vi "All Windows Out.vi"(8 "error in (no error)":errorcluster, 11 "[MDI] Parent in":refnum<class "[MDI] Parent.lvclass">) -> (0 "error out":errorcluster, 3 "[MDI] Parent out":refnum<class "[MDI] Parent.lvclass">)   [LabVIEW 2020, in "[MDI] Parent.lvlib" / "[MDI] Parent.lvclass"]
uses:
  [MDI] Parent.lvclass
  [MDI] Parent.lvclass/[MDI] Parent.ctl
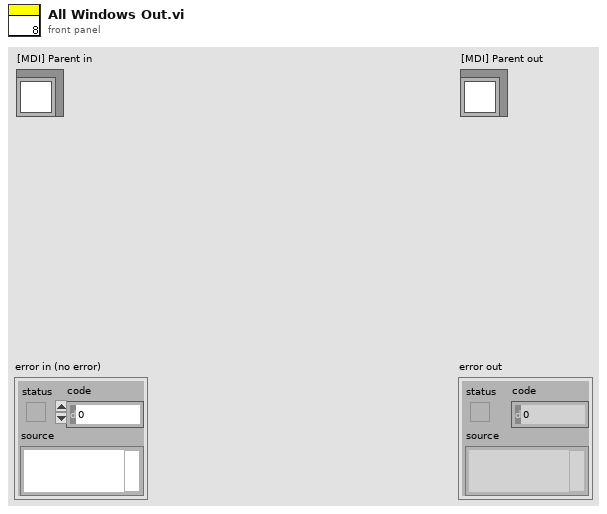
[diagram p1: front panel]
types:
  T1 = enum32{"Invalid", "Standard", "Closed", "Hidden", "Minimized", "Maximized"}
  T2 = typedef "LVRectTypeDef.ctl" = cluster{"Left":i16, "Top":i16, "Right":i16, "Bottom":i16}
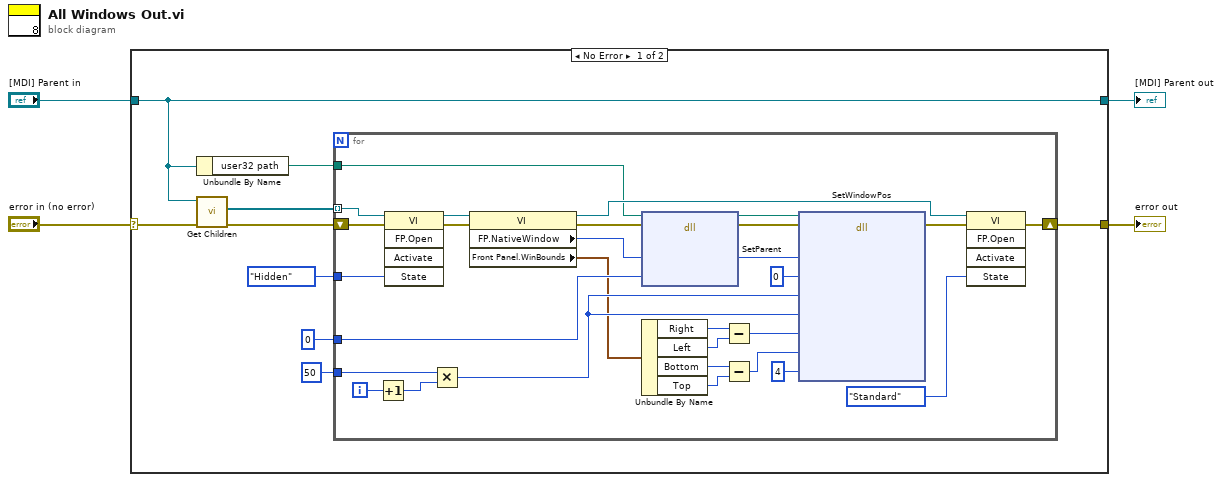
[diagram p0: block diagram]
diagram:
  n1 = case shown="No Error" "error in (no error)" {
    selector: "error in (no error)" -> [w13 w44]
    tunnel: [w7 w44] -> w3
    tunnel: [w6 w43] -> w1
    tunnel: "[MDI] Parent in" -> [w6 w43]
    frame No Error {
      n2 = Unbundle By Name(w6) -> ("user32 path"=w5:path)
      n3 = call "Get Children.vi"("error in (no error)"=w13, "[MDI] Parent in"=w6) -> ("error out"=w12:errorcluster, "all children"=w11:refnum<vi>[])  [unwired: 7 in, 1 out]
      n4 = for {
        shift-right: [w20] -> w7
        shift-left: w12 -> [w25]
        tunnel: w11 -> [w23] mode=indexing
        tunnel: u32 0 ("hWnd") -> [w42]
        tunnel: 50 -> [w37]
        tunnel: T1."Hidden" ("State") -> [w17]
        tunnel: w5 -> [w15]
        i -> [w36]
        n5 = Increment(x=w36) -> (x+1=w26:i32)
        n6 = invoke class="VI" method="FP.Open"(reference=w23, error in=w25, "State"=w17) -> (reference out=w22:refnum<vi>, error out=w24:errorcluster)  [unwired: 2 in, 3 out]
        n7 = Multiply(x=w37, y=w26) -> (x*y=w34:i32)
        n8 = property class="VI"(reference=w22, error in=w24) -> (reference out=w19:refnum<vi>, error out=w35:errorcluster, "FP.NativeWindow"=w16:u64, "Front Panel.WinBounds"=w33:T2)
        n9 = dll-call lib="user32.dll" fn="SetParent"(path in=w15, error in=w35, "child"=w16, "newParent"=w42) -> (path out=w14:path, error out=w41:errorcluster, "child"=w40:u32)  [unwired: 3 in]
        n10 = Unbundle By Name(w33) -> ("Right"=w32:i16, "Left"=w31:i16, "Bottom"=w29:i16, "Top"=w28:i16)
        n11 = Subtract(x=w32, y=w31) -> (x-y=w30:i16)
        n12 = Subtract(x=w29, y=w28) -> (x-y=w27:i16)
        n13 = dll-call lib="user32.dll" fn="SetWindowPos"(path in=w14, error in=w41, "hWnd"=w40, "hWndInsertAfter"=u32 0, "x"=w34, "y"=w34, "cx"=w30, "cy"=w27, "uFlags"=u32 4) -> (error out=w21:errorcluster)  [unwired: 9 in, 1 out]
        n14 = invoke class="VI" method="FP.Open"(reference=w19, error in=w21, "State"=T1."Standard") -> (error out=w20:errorcluster)  [unwired: 2 in, 4 out]
      }
    }
    frame Error {
    }
  }
  "error out" <- w3
  "[MDI] Parent out" <- w1
